vi "PAX_init.vi"(9 "Error In":errorcluster) -> (1 "error out":errorcluster, 2 "偏振测量仪VISA":refnum<visa-resource-name>)   [LabVIEW 2018]
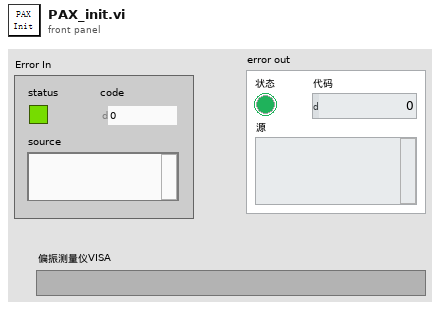
[diagram p1: front panel]
types:
  T1 = typedef "IMAQ Image.ctl" = refnum<image>
  T2 = cluster{"示波器":cluster{"Channel (0:Channel 1)":enum16{"Channel 1", "Channel 2", "Channel 3", "Channel 4"}, "电压范围":dbl, "触发电压":dbl, "时间范围":dbl, " 示波器VISA":refnum<visa-resource-name>, "时间范围 标签":u64, "电压范围 标签":u64, "触发电压 标签":u64, "输入阻抗/Ω":u64}, "光谱仪":cluster{"SpecDataReference":refnum<queue>, "grating center":dbl, "Exposure Time (s)":dbl, "是否进行详细设置":bool, " 开始通信检查":bool, "通信成功？":bool, "波长":dbl}, " 近场相机":cluster{"曝光时间/us":dbl, "模拟增益":i32, "控制套接字":i32, "IP 地址":string, " 采集套接字":i32, "  版本号":i32, "ImageData":T1, "  增益最大":i32, "  增益最小":i32, " 曝光最大":i32, " 曝光最小":i32, " 帧速":i32, " 同步切换":i32, "  曝光缩放":i32, "Camera Source":refnum<k21>, "近场X范围":dbl, "近场Y范围":dbl, "单个像元大小/um":dbl, "相机距离原点位置":dbl[], "是否测量发散角":bool, "光束类型(发散T)":bool, "聚焦透镜焦距mm":dbl}, " 偏振仪":cluster{"电压范围":u64, "触发电压":u64, "时间范围":u64, "波长范围":enum16{"可见光 400-700nm", "近红外 700-1100nm"}, "可见光偏振测量仪VISA":refnum<visa-resource-name>, "近红外偏振测量仪VISA":refnum<visa-resource-name>}, " 功率计":cluster{"通道":enum16{"Channel 1", "Channel 2"}, "工作波长":u32, "单位":u64, "时间范围":u64, "IP地址":string, "端口":u32, "是否需要散射片":bool}, "能量计":cluster{"通道":enum16{"Channel 1", "Channel 2"}, "工作波长":u32, "单位":u64, "时间范围":u64, "IP地址":string, "端口":u32, "能量计量程":enum16{"200uJ", "20uJ", "2uJ", "200nJ"}}, "电机":cluster{"Channel (0:Channel 1)":enum16{"Channel 1", "Channel 2", "Channel 3", "Channel 4"}, "电压范围":u64, "触发电压":u64, "时间范围":u64}, " 远场相机":cluster{"曝光时间":i32, "模拟增益":i32, "控制套接字":i32, "IP 地址":string, " 采集套接字":i32, "  版本号":i32, "ImageData":T1, "  增益最大":i32, "  增益最小":i32, " 曝光最大":i32, " 曝光最小":i32, " 帧速":i32, " 同步切换":i32, "  曝光缩放":i32, "ImageData B":T1, "是否远场测量":bool}}
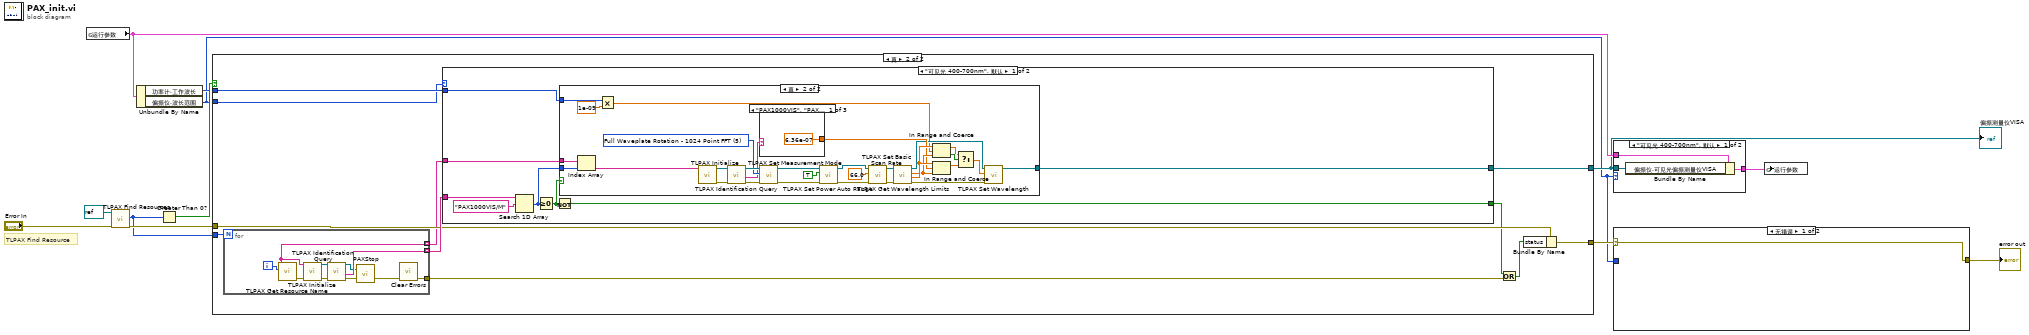
[diagram p0: block diagram]
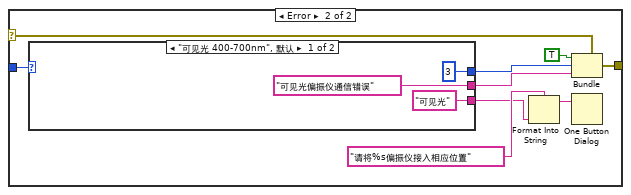
[diagram p2: hidden frame]
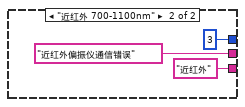
[diagram p3: hidden frame]
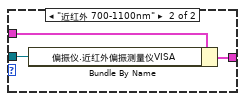
[diagram p4: hidden frame]
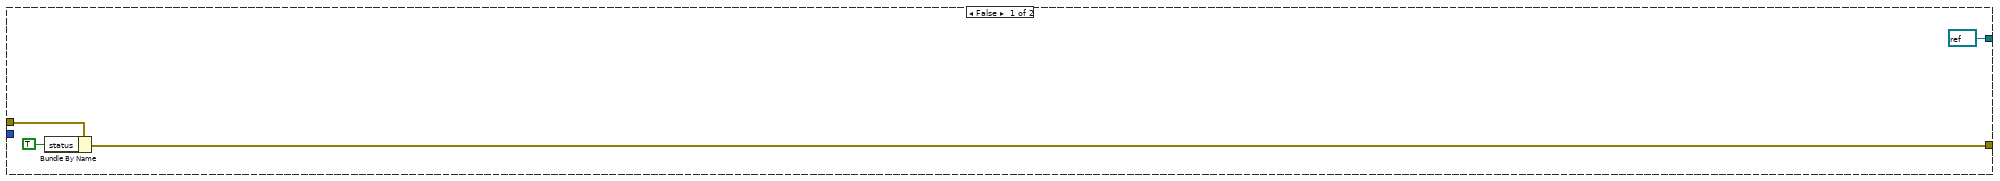
[diagram p5: hidden frame]
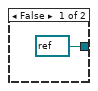
[diagram p6: hidden frame]
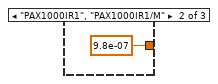
[diagram p7: hidden frame]
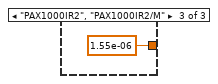
[diagram p8: hidden frame]
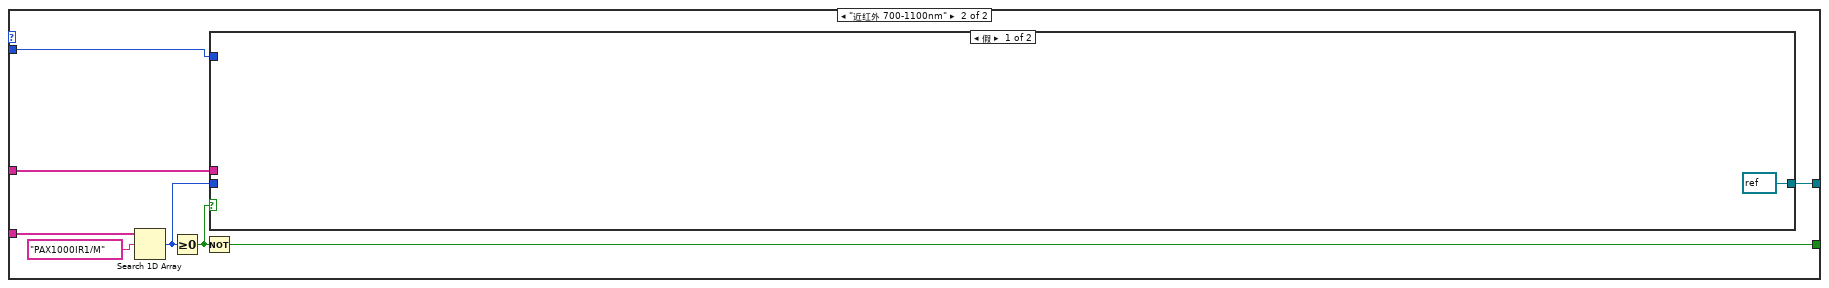
[diagram p9: hidden frame]
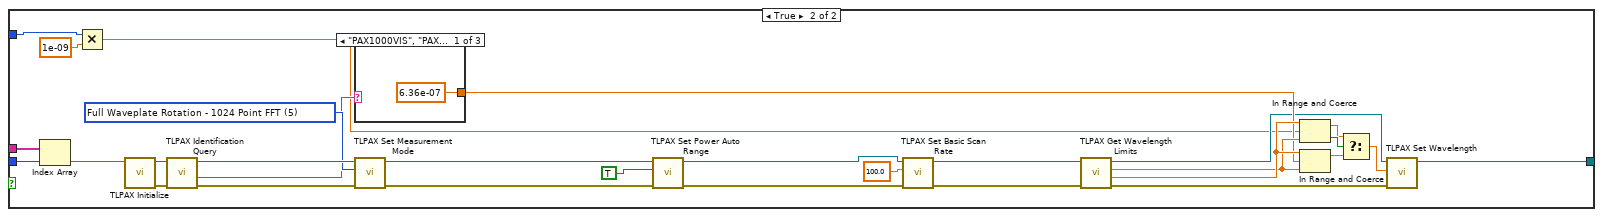
[diagram p10: hidden frame]
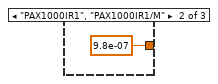
[diagram p11: hidden frame]
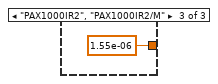
[diagram p12: hidden frame]
diagram:
  # "TLPAX Find Resource"
  n1 = global read "参数.vi" "运行参数"() -> (w9:T2)
  n2 = call <instrlib>:"TLPAX Find Resources.vi"("error in (no error)"="Error In", "instrument handle"=refnum<visa-resource-name> refnum) -> ("error out"=w6:errorcluster, "Device Count"=w4:u32)  [unwired: 7 in, 1 out]
  n3 = Unbundle By Name(w9) -> ("功率计.工作波长"=w5:u32, "偏振仪.波长范围"=w2:enum16{"可见光 400-700nm", "近红外 700-1100nm"})
  n4 = Greater Than 0?(x=w4) -> (x > 0?=w10:bool)
  n5 = case shown="真" w10 {
    tunnel: w6 -> [w16 w25]
    tunnel: w5 -> [_ w21]
    tunnel: [refnum<visa-resource-name> refnum ("instrument handle") w22] -> w7
    tunnel: [w14 w24] -> w3
    tunnel: w2 -> [_ w17]
    tunnel: w4 -> [_ w26]
    frame False {
      n6 = Bundle By Name(cluster=w16, "status"=TRUE) -> (w14:errorcluster)
    }
    frame True {
      n7 = for {
        N: w26 -> [_]
        tunnel: [w117] -> w27 mode=indexing
        tunnel: [w114] -> w23 mode=indexing
        tunnel: [w112] -> w18
        i -> [w118]
        n8 = call <instrlib>:"TLPAX Get Resource Name.vi"("Index (0)"=w118) -> ("error out"=w119:errorcluster, "Resource Name"=w114:string)  [unwired: 8 in, 1 out]
        n9 = call <instrlib>:"TLPAX Initialize.vi"("error in (no error)"=w119, "resource name"=w114) -> ("error out"=w120:errorcluster, "instrument handle out"=w121:refnum<visa-resource-name>)  [unwired: 8 in]
        n10 = call <instrlib>:"TLPAX Identification Query.vi"("error in (no error)"=w120, "instrument handle"=w121) -> ("error out"=w115:errorcluster, "Device Name"=w117:string, "instrument handle out"=w116:refnum<visa-resource-name>)  [unwired: 4 in, 3 out]
        n11 = call "PAXStop.vi"("error in"=w115, "VISA 输入"=w116) -> ("error out"=w113:errorcluster)  [unwired: 1 in]
        n12 = call <vilib>:"Clear Errors.vi"("error in (no error)"=w113) -> ("error out"=w112:errorcluster)  [unwired: 5 in, 1 out]
      }
      n13 = case shown="\"可见光 400-700nm\", 默认" w17 {
        tunnel: w27 -> [w34 w75]
        tunnel: [w32 w74] -> w19
        tunnel: w23 -> [w31 w73]
        tunnel: [w29 w71] -> w22
        tunnel: w21 -> [w28 w70]
        frame "可见光 400-700nm", Default {
          n14 = Search 1D Array(1D array=w34, element="PAX1000VIS/M" ("元素")) -> (index of element=w30:i32)  [unwired: 1 in]
          n15 = Greater Or Equal To 0?(x=w30) -> (x >= 0?=w33:bool)
          n16 = Not(x=w33) -> (.not. x?=w32:bool)
          n17 = case shown="真" w33 {
            tunnel: w31 -> [_ w66]
            tunnel: w30 -> [_ w65]
            tunnel: [refnum<visa-resource-name> refnum ("instrument handle out") w38] -> w29
            tunnel: w28 -> [_ w37]
            frame False {
            }
            frame True {
              w60 = 5 items=["Idle", "Half Waveplate Rotation - 512 Point FFT", "Half Waveplate Rotation - 1024 Point FFT", "Half Waveplate Rotation - 2048 Point FFT", "Full Waveplate Rotation - 512 Point FFT", "Full Waveplate Rotation - 1024 Point FFT", "Full Waveplate Rotation - 2048 Point FFT", "Double Waveplate Rotation - 512 Point FFT", "Double Waveplate Rotation - 1024 Point FFT", "Double Waveplate Rotation - 2048 Point FFT"] ("Operation Mode")
              n18 = Index Array(array=w66, index=w65) -> (element=w39:string)
              n19 = Multiply(x=w37, y=1e-09) -> (x*y=w40:dbl)
              n20 = call <instrlib>:"TLPAX Initialize.vi"("resource name"=w39) -> ("error out"=w64:errorcluster, "instrument handle out"=w63:refnum<visa-resource-name>)  [unwired: 9 in]
              n21 = call <instrlib>:"TLPAX Identification Query.vi"("error in (no error)"=w64, "instrument handle"=w63) -> ("error out"=w62:errorcluster, "Device Name"=w53:string, "instrument handle out"=w61:refnum<visa-resource-name>)  [unwired: 4 in, 3 out]
              n22 = case shown="\"PAX1000VIS\", \"PAX1000VIS/M\", 默认" w53 {
                tunnel: [6.36e-07 ("Wavelength") 9.8e-07 ("Wavelength") 1.55e-06 ("Wavelength")] -> w46
                frame "PAX1000VIS", "PAX1000VIS/M", Default {
                }
                frame "PAX1000IR1", "PAX1000IR1/M" {
                }
                frame "PAX1000IR2", "PAX1000IR2/M" {
                }
              }
              n23 = call <instrlib>:"TLPAX Set Measurement Mode.vi"("error in (no error)"=w62, "Mode (Double Waveplate Rotation - 2048 Point FFT)"=w60, "instrument handle"=w61) -> ("error out"=w59:errorcluster, "instrument handle out"=w58:refnum<visa-resource-name>)  [unwired: 7 in]
              n24 = call <instrlib>:"TLPAX Set Power Auto Range.vi"("error in (no error)"=w59, "Autorange (On)"=TRUE ("Autorange"), "instrument handle"=w58) -> ("error out"=w56:errorcluster, "instrument handle out"=w55:refnum<visa-resource-name>)  [unwired: 7 in]
              n25 = call <instrlib>:"TLPAX Set Basic Scan Rate.vi"("error in (no error)"=w56, "Basic Scan Rate"=66.0, "instrument handle"=w55) -> ("error out"=w49:errorcluster, "instrument handle out"=w50:refnum<visa-resource-name>)  [unwired: 7 in]
              n26 = call <instrlib>:"TLPAX Get Wavelength Limits.vi"("error in (no error)"=w49, "instrument handle"=w50) -> ("error out"=w52:errorcluster, "Maximum"=w48:dbl, "Minimum"=w47:dbl, "instrument handle out"=w42:refnum<visa-resource-name>)  [unwired: 6 in]
              n27 = In Range and Coerce(upper limit=w48, x=w40, lower limit=w47) -> (coerced(x)=w44:dbl, In Range?=w45:bool)
              n28 = In Range and Coerce(upper limit=w48, x=w46, lower limit=w47) -> (coerced(x)=w51:dbl)  [unwired: 1 out]
              n29 = Select(t=w44, s=w45, f=w51) -> (s? t:f=w43:dbl)
              n30 = call <instrlib>:"TLPAX Set Wavelength.vi"("error in (no error)"=w52, "Wavelength"=w43, "instrument handle"=w42) -> ("instrument handle out"=w38:refnum<visa-resource-name>)  [unwired: 7 in, 1 out]
            }
          }
        }
        frame "近红外 700-1100nm" {
          n31 = Search 1D Array(1D array=w75, element="PAX1000IR1/M" ("元素")) -> (index of element=w72:i32)  [unwired: 1 in]
          n32 = Greater Or Equal To 0?(x=w72) -> (x >= 0?=w76:bool)
          n33 = Not(x=w76) -> (.not. x?=w74:bool)
          n34 = case shown="假" w76 {
            tunnel: w73 -> [_ w83]
            tunnel: w72 -> [_ w82]
            tunnel: [refnum<visa-resource-name> refnum ("instrument handle out") w80] -> w71
            tunnel: w70 -> [_ w79]
            frame False {
            }
            frame True {
              w104 = 5 items=["Idle", "Half Waveplate Rotation - 512 Point FFT", "Half Waveplate Rotation - 1024 Point FFT", "Half Waveplate Rotation - 2048 Point FFT", "Full Waveplate Rotation - 512 Point FFT", "Full Waveplate Rotation - 1024 Point FFT", "Full Waveplate Rotation - 2048 Point FFT", "Double Waveplate Rotation - 512 Point FFT", "Double Waveplate Rotation - 1024 Point FFT", "Double Waveplate Rotation - 2048 Point FFT"] ("Operation Mode")
              n35 = Index Array(array=w83, index=w82) -> (element=w81:string)
              n36 = Multiply(x=w79, y=1e-09) -> (x*y=w84:dbl)
              n37 = call <instrlib>:"TLPAX Initialize.vi"("resource name"=w81) -> ("error out"=w108:errorcluster, "instrument handle out"=w107:refnum<visa-resource-name>)  [unwired: 9 in]
              n38 = call <instrlib>:"TLPAX Identification Query.vi"("error in (no error)"=w108, "instrument handle"=w107) -> ("error out"=w106:errorcluster, "Device Name"=w97:string, "instrument handle out"=w105:refnum<visa-resource-name>)  [unwired: 4 in, 3 out]
              n39 = case shown="\"PAX1000VIS\", \"PAX1000VIS/M\", 默认" w97 {
                tunnel: [6.36e-07 ("Wavelength") 9.8e-07 ("Wavelength") 1.55e-06 ("Wavelength")] -> w90
                frame "PAX1000VIS", "PAX1000VIS/M", Default {
                }
                frame "PAX1000IR1", "PAX1000IR1/M" {
                }
                frame "PAX1000IR2", "PAX1000IR2/M" {
                }
              }
              n40 = call <instrlib>:"TLPAX Set Measurement Mode.vi"("error in (no error)"=w106, "Mode (Double Waveplate Rotation - 2048 Point FFT)"=w104, "instrument handle"=w105) -> ("error out"=w103:errorcluster, "instrument handle out"=w102:refnum<visa-resource-name>)  [unwired: 7 in]
              n41 = call <instrlib>:"TLPAX Set Power Auto Range.vi"("error in (no error)"=w103, "Autorange (On)"=TRUE ("Autorange"), "instrument handle"=w102) -> ("error out"=w100:errorcluster, "instrument handle out"=w99:refnum<visa-resource-name>)  [unwired: 7 in]
              n42 = call <instrlib>:"TLPAX Set Basic Scan Rate.vi"("error in (no error)"=w100, "Basic Scan Rate"=100.0, "instrument handle"=w99) -> ("error out"=w93:errorcluster, "instrument handle out"=w94:refnum<visa-resource-name>)  [unwired: 7 in]
              n43 = call <instrlib>:"TLPAX Get Wavelength Limits.vi"("error in (no error)"=w93, "instrument handle"=w94) -> ("error out"=w96:errorcluster, "Maximum"=w92:dbl, "Minimum"=w91:dbl, "instrument handle out"=w86:refnum<visa-resource-name>)  [unwired: 6 in]
              n44 = In Range and Coerce(upper limit=w92, x=w84, lower limit=w91) -> (coerced(x)=w88:dbl, In Range?=w89:bool)
              n45 = In Range and Coerce(upper limit=w92, x=w90, lower limit=w91) -> (coerced(x)=w95:dbl)  [unwired: 1 out]
              n46 = Select(t=w88, s=w89, f=w95) -> (s? t:f=w87:dbl)
              n47 = call <instrlib>:"TLPAX Set Wavelength.vi"("error in (no error)"=w96, "Wavelength"=w87, "instrument handle"=w86) -> ("instrument handle out"=w80:refnum<visa-resource-name>)  [unwired: 7 in, 1 out]
            }
          }
        }
      }
      n48 = Or(x=w19, y=w18) -> (x .or. y?=w20:bool)
      n49 = Bundle By Name(cluster=w25, "status"=w20) -> (w24:errorcluster)
    }
  }
  "偏振测量仪VISA" <- w7
  n50 = case shown="\"可见光 400-700nm\", 默认" w2 {
    tunnel: w9 -> [w124 w127]
    tunnel: [w123 w126] -> w8
    tunnel: w7 -> [w122 w125]
    frame "可见光 400-700nm", Default {
      n51 = Bundle By Name(cluster=w124, "偏振仪.可见光偏振测量仪VISA"=w122) -> (w123:T2)
    }
    frame "近红外 700-1100nm" {
      n52 = Bundle By Name(cluster=w127, "偏振仪.近红外偏振测量仪VISA"=w125) -> (w126:T2)
    }
  }
  n53 = case shown="无错误" w3 {
    selector: w3 -> [w128 w136]
    tunnel: w2 -> [_ w137]
    tunnel: [w128 w132] -> w1
    frame No Error {
    }
    frame Error {
      n54 = case shown="\"可见光 400-700nm\", 默认" w137 {
        tunnel: [3 ("code") 3 ("code")] -> w134
        tunnel: ["可见光偏振仪通信错误" ("source") "近红外偏振仪通信错误" ("source")] -> w133
        tunnel: ["可见光" "近红外"] -> w130
        frame "可见光 400-700nm", Default {
        }
        frame "近红外 700-1100nm" {
        }
      }
      n55 = Format Into String(format string="请将%s偏振仪接入相应位置" ("格式字符串"), w130) -> (resulting string=w129:string)  [unwired: 2 in, 1 out]
      n56 = Bundle(cluster=w136, "status"=TRUE, "code"=w134, "source"=w133) -> (w132:errorcluster)
      n57 = One Button Dialog(message=w129) -> ()  [unwired: 1 in, 1 out]
    }
  }
  "error out" <- w1
  n58 = global write "参数.vi" "运行参数"(w8) -> ()
